vi "Strip brackets with Option.vi"(1 "TYPE":T1(ring)=enum."0x5B5D - []", 3 "trimmed string in":string) -> (0 "trimmed string out":string)   [LabVIEW 2017, in "API String Arguments Support.lvlib"]
uses:
  API String Arguments Support.lvlib
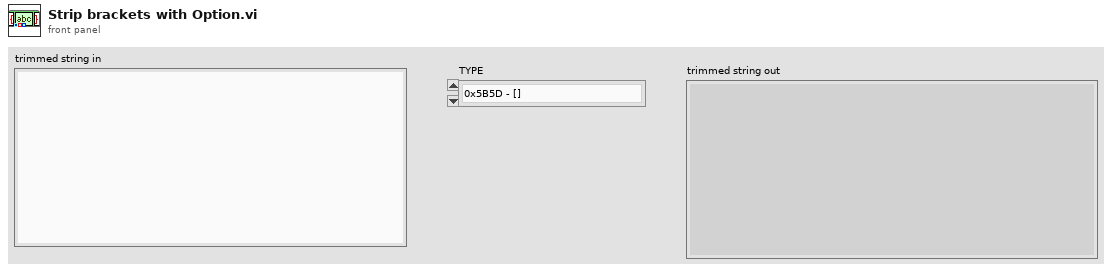
[diagram p1: front panel]
types:
  T1 = enum16{"0x2829 - ()", "0x5B5D - []", "0x7B7D - {}"}
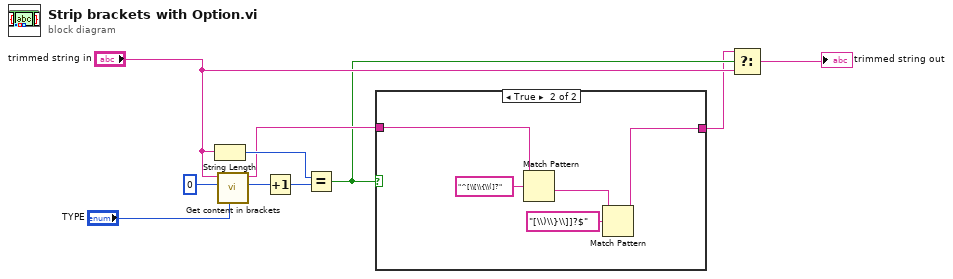
[diagram p0: block diagram]
diagram:
  n1 = String Length(string="trimmed string in") -> (length=w6:i32)
  n2 = call "Get content in brackets.vi"("TYPE"="TYPE", "start"=0, "String in"="trimmed string in") -> ("index out"=w7:i32, "String out"=w5:string)  [unwired: 7 in]
  n3 = Increment(x=w7) -> (x+1=w4:i32)
  n4 = Equal?(x=w6, y=w4) -> (x = y?=w3:bool)
  n5 = case shown="True" w3 {
    tunnel: [w11 w16] -> w2
    tunnel: w5 -> [w11 w14]
    frame False {
    }
    frame True {
      n6 = Match Pattern(string=w14, regular expression="^[\\[\\{\\(]?") -> (after substring=w13:string)  [unwired: 1 in, 3 out]
      n7 = Match Pattern(string=w13, regular expression="[\\)\\}\\]]?$") -> (before substring=w16:string)  [unwired: 1 in, 3 out]
    }
  }
  n8 = Select(t=w2, s=w3, f="trimmed string in") -> (s? t:f=→"trimmed string out":string)
